vi "Join Strings in node-path.vi"(7 "Glue":string=".", 10 "Array of Strings":string[](array[string]), 11 "Prefix":string="$") -> (3 "Result":string)   [LabVIEW 2018, in "ClientMessaging.lvlib"]
doc: "Join the elements of the array together separated by the <b>glue</b> and with <b>prefix</b> at the start.\n\nUSed to construct a $.name.name.name path for parsing JSON with JSONtext"
uses:
  ClientMessaging.lvlib
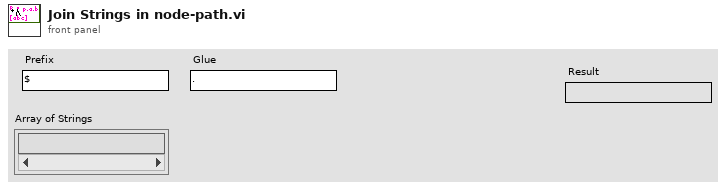
[diagram p1: front panel]
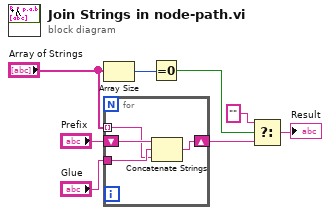
[diagram p0: block diagram]
diagram:
  n1 = Array Size(array="Array of Strings") -> (size(s)=w5:i32)
  n2 = for {
    shift-right: [w9] -> w3
    shift-left: "Prefix" -> [w12]
    tunnel: "Glue" -> [w11]
    tunnel: "Array of Strings" -> [w10] mode=indexing
    n3 = Concatenate Strings(w12, w11, w10) -> (w9:string)
  }
  n4 = Equal To 0?(x=w5) -> (x = 0?=w4:bool)
  n5 = Select(t="", s=w4, f=w3) -> (s? t:f=→"Result":string)
